vi "test-tagRouter.vi"() -> ()   [LabVIEW 2020]
uses:
  9c45d527-4fff-4982-a2e1-f8d778b02ec9.vi
  <userlib>/_NEVSTOP/Communicable State Machine(CSM)/AdvanceAPI/CSM - Break Down Multiple States String.vi
  <userlib>/_NEVSTOP/Communicable State Machine(CSM)/AdvanceAPI/CSM - Compact Multiple States.vi
  <userlib>/_NEVSTOP/Communicable State Machine(CSM)/AdvanceAPI/CSM - Revert Arguments-Safe String.vi
  <userlib>/_NEVSTOP/Communicable State Machine(CSM)/_Shared/Trim Single-line Text.vi
  <userlib>/_NEVSTOP/Communicable State Machine(CSM)/AdvanceAPI/CSM - Make String Arguments Safe.vi
  <userlib>/_NEVSTOP/Communicable State Machine(CSM)/AdvanceAPI/CSM - Keywords.vi
  <userlib>/_NEVSTOP/Communicable State Machine(CSM)/Utility/CSM Data Type String.vi
  <userlib>/_NEVSTOP/Communicable State Machine(CSM)/addons/MassData-Parameter/_support/FGV-MassData(lvlibp).vi
  CSM-TagRouter.lvlib
  <userlib>/_NEVSTOP/Communicable State Machine(CSM)/Communicable State Machine.lvlib
  <userlib>/_NEVSTOP/TagDB/TagDB.lvlib
panel:
  out "Data":variant[](array[variant])
  out "names":string[](array[string])
  in  "WaveformGen Settings":T1(array[cluster])=[{"sampling info"={"Fs"=1000.0, "#s"=1000.0}, "phase"=0.0, "amplitude"=1.0, "frequency"=10.0, "range"=1.0, "Type"=enum."Sine", "Waveform Name"="Waveform 0"}, {"sampling info"={"Fs"=1000.0, "#s"=1000.0}, "phase"=0.0, "amplitude"=1.0, "frequency"=10.0, "range"=1.0, "Type"=enum."Triangle", "Waveform Name"="Waveform 1"}, {"sampling info"={"Fs"=1000.0, "#s"=1000.0}, "phase"=0.0, "amplitude"=1.0, "frequency"=10.0, "range"=1.0, "Type"=enum."Sawtooth", "Waveform Name"="Waveform 2"}, {"sampling info"={"Fs"=1000.0, "#s"=1000.0}, "phase"=0.0, "amplitude"=1.0, "frequency"=10.0, "range"=1.0, "Type"=enum."Square", "Waveform Name"="Waveform 3"}]
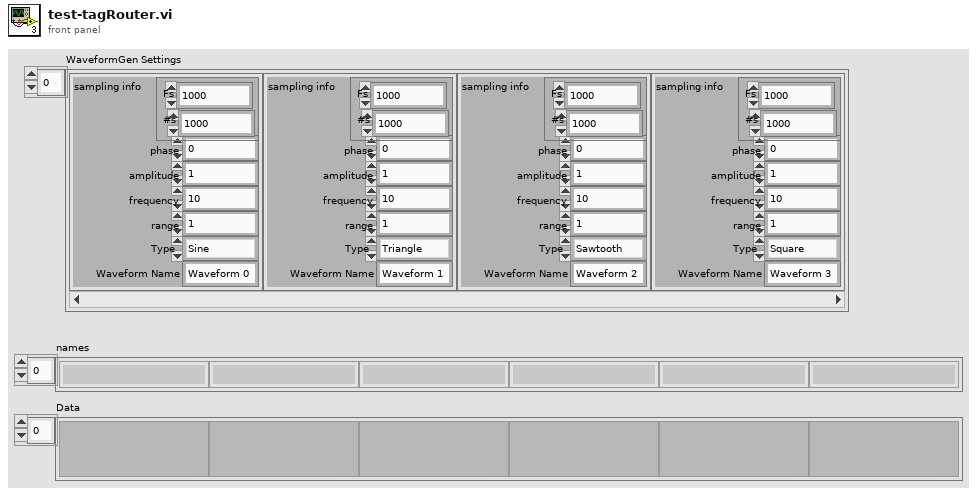
[diagram p1: front panel]
types:
  T1 = cluster{"sampling info":cluster{"Fs":dbl, "#s":dbl}, "phase":dbl, "amplitude":dbl, "frequency":dbl, "range":dbl, "Type":enum16{"Sine", "Triangle", "Sawtooth", "Square"}, "Waveform Name":string}[]
  T2 = enum32{"Invalid", "Standard", "Closed", "Hidden", "Minimized", "Maximized"}
  T3 = enum32{"invalid app kind", "Development System", "Run Time System", "Student Edition", "Embedded LabVIEW", "Evaluation", "Custom"}
  T4 = typedef "Communicable State Machine.lvlib/_CSM_Response Source Message.ctl" = cluster{"‘State":string, "’Arguments":string, "’Error":errorcluster}
  T5 = cluster{"Current VI Reference":refnum<vi>, "Close Panel on Exit?":bool}
  T6 = cluster{"Core":cluster{"Current VI Reference":refnum<vi>, "Close Panel on Exit?":bool}, "Your Boolean data":bool, "Your string data":string}
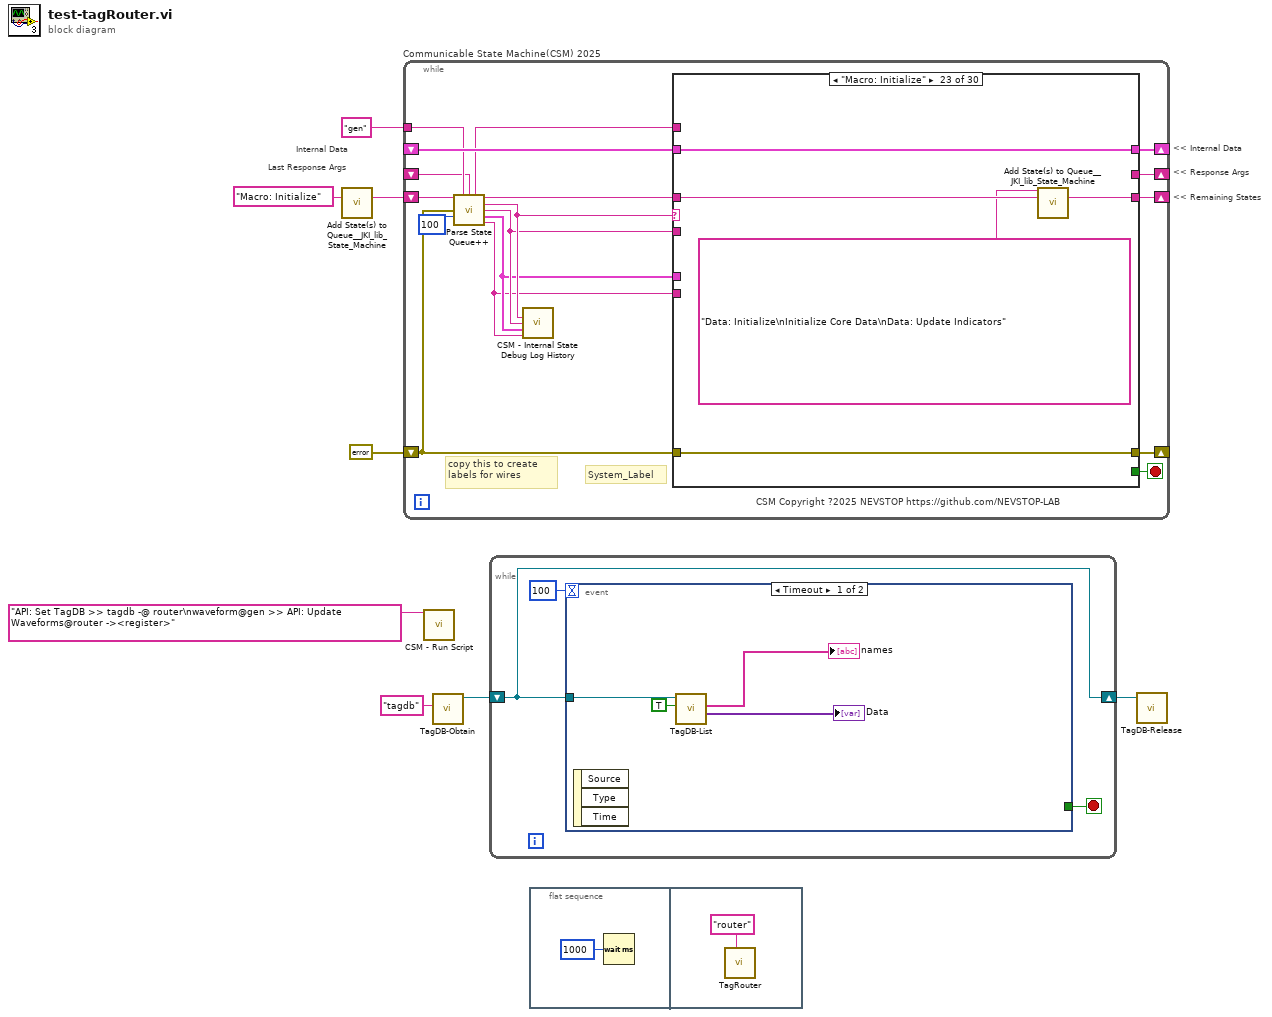
[diagram p0: block diagram]
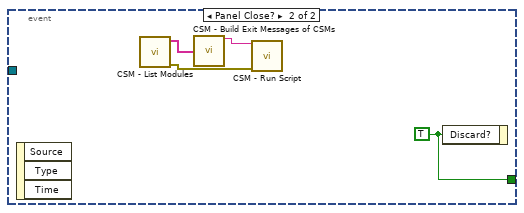
[diagram p2: hidden frame]
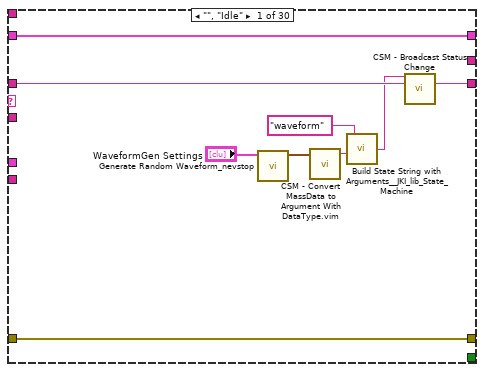
[diagram p3: hidden frame]
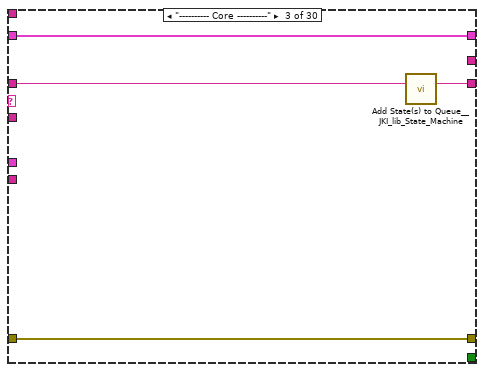
[diagram p5: hidden frame]
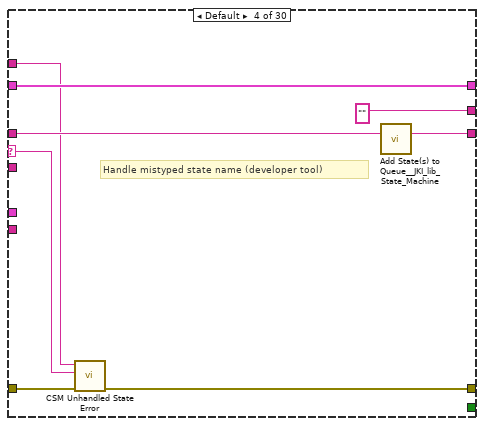
[diagram p6: hidden frame]
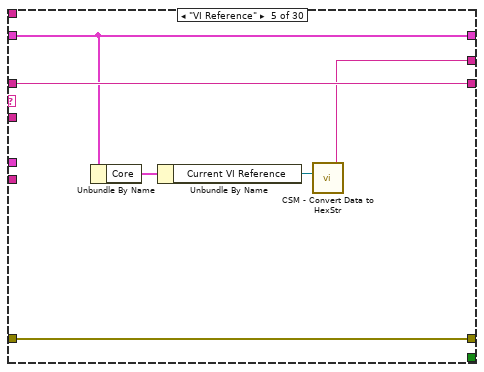
[diagram p7: hidden frame]
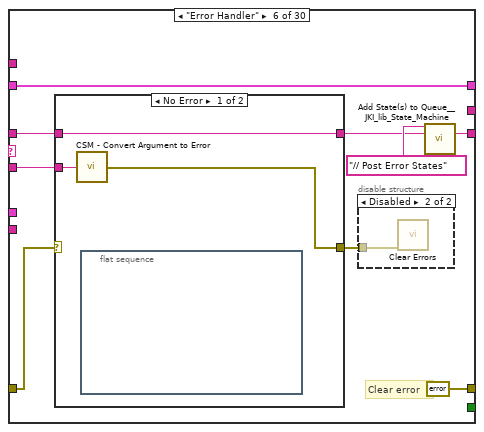
[diagram p8: hidden frame]
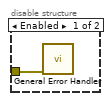
[diagram p9: hidden frame]
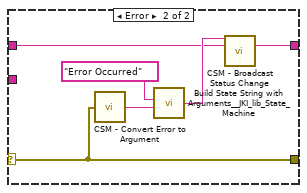
[diagram p10: hidden frame]
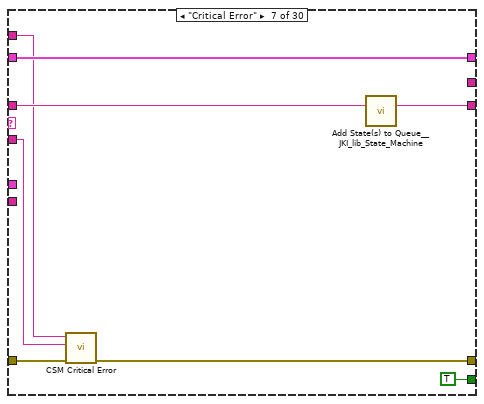
[diagram p11: hidden frame]
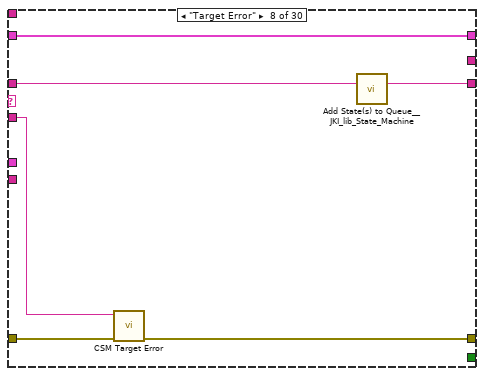
[diagram p12: hidden frame]
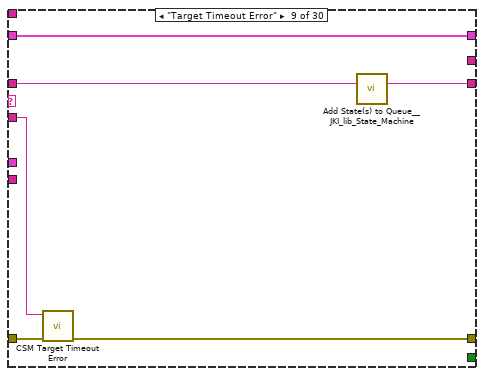
[diagram p13: hidden frame]
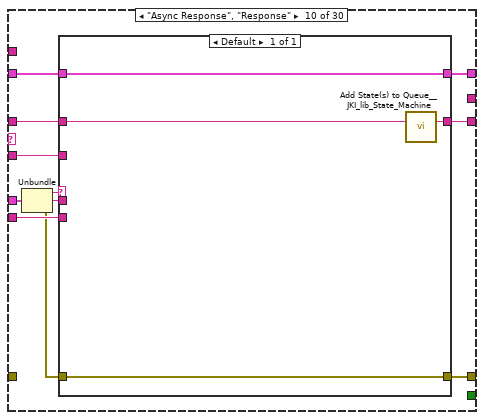
[diagram p14: hidden frame]
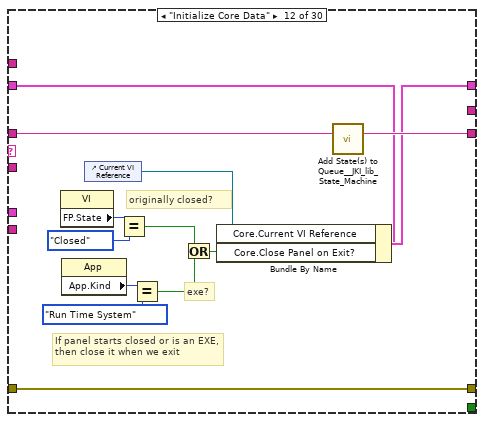
[diagram p16: hidden frame]
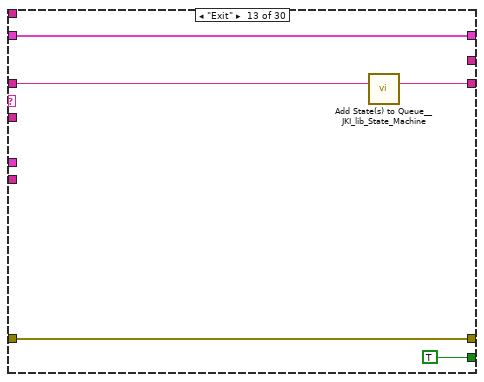
[diagram p17: hidden frame]
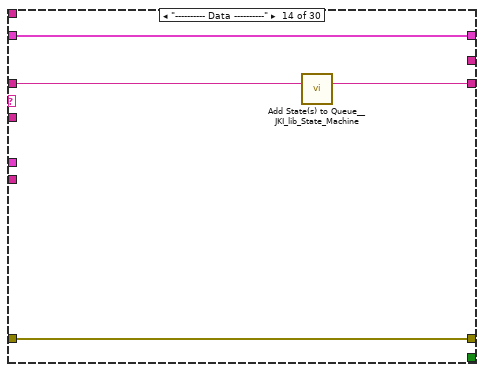
[diagram p18: hidden frame]
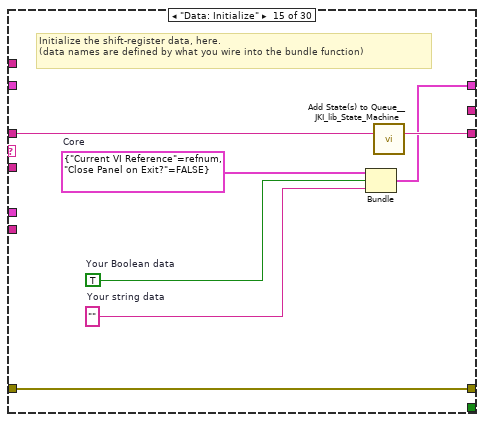
[diagram p19: hidden frame]
diagram:
  # "Last Response Args"
  # "Internal Data"
  # "<< Internal Data"
  # "<< Response Args"
  # "<< Remaining States"
  n1 = call <vilib>:"Add State(s) to Queue__JKI_lib_State_Machine.vi"("State(s) in (\"\")"="Macro: Initialize" ("Init State(\"Macro: Initialize\")")) -> ("States Out"=w5:string)  [unwired: 14 in]
  n2 = while "Communicable State Machine(CSM) 2025" {
    shift-right: [w20] -> _
    shift-left: _ -> [w19]
    shift-right: [w23] -> _
    shift-left: errorcluster {"status"=FALSE, "code"=0, "source"=""} ("error out") -> [w18]
    shift-right: [w22] -> _
    shift-left: w5 -> [w24]
    tunnel: "gen" ("Name (\"\" to Use UUID)") -> [w16]
    shift-right: [w17] -> _
    shift-left: _ -> [w10]
    stop <- w21 stop-if-true
    # "copy this to create labels for wires"
    # "System_Label"
    # "CSM Copyright ?2025 NEVSTOP https://github.com/NEVSTOP-LAB"
    n3 = call <userlib>:"Parse State Queue++.vi"("State Queue"=w24, "Name (\"\" to Use UUID)"=w16, "Response Arguments"=w10, "Previous Error"=w18, "Dequeue (1 ms)"=100 ("Timeout")) -> ("Name Used"=w11:string, "Remaining States"=w25:string, "Current State"=w15:string, "Arguments"=w14:string, "Additional Information"=w13:T4, "Source CSM"=w12:string)  [unwired: 5 in]
    n4 = call <userlib>:"CSM - Internal State Debug Log History.vi"("State"=w15, "Arguments (\"\")"=w14, ">> Response Source Message >>"=w13, "Source (\"\")"=w12) -> ()  [unwired: 11 in, 1 out]
    n5 = case shown="\"Macro: Initialize\"" w15 {
      selector: w15 -> [_ _ _ w44 _ _ _ _ _ _ _ _ _ _ _ _ _ _ _ _ _ _ _ _ _ _ _ _ _ _]
      tunnel: w25 -> [w31 w36 w41 w48 w54 w60 w81 w87 w93 w101 w112 w126 w131 w135 w142 w144 w151 w155 w159 w165 w180 w249 w254 w261 w263 w267 w272 w279 w283 w287]
      tunnel: w14 -> [_ _ _ _ _ w59 w77 w86 w91 w100 _ _ _ _ _ _ _ _ _ w160 w174 _ _ _ _ _ w270 _ _ _]
      tunnel: w19 -> [w32 w35 w38 w46 w53 w63 w82 w88 w94 w103 w111 w119 w129 w132 _ w143 w146 w152 w157 w163 w176 w246 w251 w258 w262 w266 w271 w276 w280 w284]
      tunnel: [w33 w37 w39 w42 w55 errorcluster {"status"=FALSE, "code"=0, "source"=""} ("error out") w78 w84 w90 w106 w113 w123 w128 w133 w139 w145 w147 w153 w156 w161 w177 w247 w252 w259 w264 w268 w273 w277 w281 w285] -> w23
      tunnel: w18 -> [w33 w37 w39 w49 w55 w61 w83 w85 w92 _ w113 w123 w128 w133 w139 w145 w148 w153 w156 w162 w178 w247 w252 w259 w264 w268 w273 w277 w281 w285]
      tunnel: [w34 w36 w40 w47 w54 w56 w80 w89 w95 w102 w112 w125 w130 w134 w141 w144 w150 w154 w158 w164 w179 w248 w253 w260 w263 w267 w272 w278 w282 w286] -> w22
      tunnel: [_ _ _ _ _ _ TRUE _ _ _ _ _ TRUE _ _ _ _ _ _ _ _ _ _ _ _ _ _ _ _ _] -> w21
      tunnel: [w32 w35 w38 w46 w53 w63 w82 w88 w94 w104 w111 w124 w129 w132 w140 w143 w146 w152 w157 w163 w176 w246 w251 w258 w262 w266 w271 w276 w280 w284] -> w20
      tunnel: w12 -> [_ _ _ _ _ _ _ _ _ w98 _ _ _ _ _ _ _ _ _ _ _ _ _ _ _ _ _ _ _ _]
      tunnel: w13 -> [_ _ _ _ _ _ _ _ _ w105 _ _ _ _ _ _ _ _ _ _ _ _ _ _ _ _ _ _ _ _]
      tunnel: [_ _ _ "" w50 _ _ _ _ _ _ _ _ _ _ _ _ _ _ _ _ _ _ _ _ "API1 Response" w269 _ _ _] -> w17
      tunnel: w11 -> [_ _ _ w43 _ _ w76 _ _ _ _ _ _ _ _ _ _ _ _ _ _ _ _ _ _ _ _ _ _ _]
      frame "", "Idle" {
        n6 = call <userlib>:"Generate Random Waveform_nevstop.vi"("WaveformGen Settings"="WaveformGen Settings") -> ("Waveforms"=w29:waveform(dbl)[])  [unwired: 9 in, 1 out]
        n7 = call "CSM - Convert MassData to Argument With DataType.vim"("Data"=w29) -> ("MassData Argument"=w28:string)  [unwired: 7 in, 1 out]
        n8 = call <vilib>:"Build State String with Arguments__JKI_lib_State_Machine.vi"("Arguments (\"\")"=w28, "State"="waveform") -> ("State with Arguments"=w26:string)  [unwired: 4 in]
        n9 = call <userlib>:"CSM - Broadcast Status Change.vi"("Status With Arguments"=w26, "State Queue"=w31) -> ("Remaining States"=w34:string)  [unwired: 13 in]
      }
      frame "CSM Documentation" {
      }
      frame "---------- Core ----------" {
        n10 = call <vilib>:"Add State(s) to Queue__JKI_lib_State_Machine.vi"("State(s) in (\"\")"=w41) -> ("States Out"=w40:string)  [unwired: 14 in]
      }
      frame Default {
        # "Handle mistyped state name (developer tool)"
        n11 = call <userlib>:"CSM Unhandled State Error.vi"("error in (no error)"=w49, "Undefined State"=w44, "CSM Name"=w43) -> ("error out"=w42:errorcluster)  [unwired: 8 in]
        n12 = call <vilib>:"Add State(s) to Queue__JKI_lib_State_Machine.vi"("State(s) in (\"\")"=w48) -> ("States Out"=w47:string)  [unwired: 14 in]
      }
      frame "VI Reference" {
        n13 = Unbundle By Name(w53) -> ("Core"=w52:T5)
        n14 = Unbundle By Name(w52) -> ("Current VI Reference"=w51:refnum<vi>)
        n15 = call <userlib>:"CSM - Convert Data to HexStr.vi"("Variant"=w51) -> ("HEX String (0-9,A-F)"=w50:string)  [unwired: 8 in]
      }
      frame "Error Handler" {
        # "Clear error"
        n16 = case shown="No Error" w61 {
          selector: w61 -> [_ w70]
          tunnel: [w69 w72] -> w57
          tunnel: w60 -> [w69 w71]
          tunnel: w59 -> [w68 _]
          tunnel: [w67 w70] -> w62
          frame No Error {
            n17 = call <userlib>:"CSM - Convert Argument to Error.vi"("Argument"=w68) -> ("Error"=w67:errorcluster)  [unwired: 4 in]
            n18 = flat-sequence {
              frame #0 {
              }
            }
          }
          frame Error {
            n19 = call <userlib>:"CSM - Convert Error to Argument.vi"("Error"=w70) -> ("Argument"=w74:string)  [unwired: 4 in]
            n20 = call <vilib>:"Build State String with Arguments__JKI_lib_State_Machine.vi"("Arguments (\"\")"=w74, "State"="Error Occurred" ("Status with Arguments")) -> ("State with Arguments"=w73:string)  [unwired: 4 in]
            n21 = call <userlib>:"CSM - Broadcast Status Change.vi"("Status With Arguments"=w73, "State Queue"=w71) -> ("Remaining States"=w72:string)  [unwired: 13 in]
          }
        }
        n22 = disable-structure shown="Disabled" {
          disable-tunnel: w62 -> [w65 w66]
          frame Enabled {
            n23 = call <vilib>:"General Error Handler.vi"("error in (no error)"=w65) -> ()  [unwired: 10 in, 5 out]
          }
          frame Disabled {
            n24 = call <vilib>:"Clear Errors.vi"("error in (no error)"=w66) -> ()  [unwired: 5 in, 2 out]
          }
        }
        n25 = call <vilib>:"Add State(s) to Queue__JKI_lib_State_Machine.vi"("State(s) in Front (\"\")"="// Post Error States", "State(s) in (\"\")"=w57) -> ("States Out"=w56:string)  [unwired: 13 in]
      }
      frame "Critical Error" {
        n26 = call <userlib>:"CSM Critical Error.vi"("error in (no error)"=w83, "Arugments (As Reason)"=w77, "CSM Name"=w76) -> ("error out"=w78:errorcluster)  [unwired: 8 in]
        n27 = call <vilib>:"Add State(s) to Queue__JKI_lib_State_Machine.vi"("State(s) in (\"\")"=w81) -> ("States Out"=w80:string)  [unwired: 14 in]
      }
      frame "Target Error" {
        n28 = call <userlib>:"CSM Target Error.vi"("error in (no error)"=w85, "Arguments (As CSM Name)"=w86) -> ("error out"=w84:errorcluster)  [unwired: 9 in]
        n29 = call <vilib>:"Add State(s) to Queue__JKI_lib_State_Machine.vi"("State(s) in (\"\")"=w87) -> ("States Out"=w89:string)  [unwired: 14 in]
      }
      frame "Target Timeout Error" {
        n30 = call <userlib>:"CSM Target Timeout Error.vi"("error in (no error)"=w92, "Arguments (As CSM Name)"=w91) -> ("error out"=w90:errorcluster)  [unwired: 9 in]
        n31 = call <vilib>:"Add State(s) to Queue__JKI_lib_State_Machine.vi"("State(s) in (\"\")"=w93) -> ("States Out"=w95:string)  [unwired: 14 in]
      }
      frame "Async Response", "Response" {
        n32 = Unbundle(w105) -> ("‘State"=w99:string, "’Arguments"=w97:string, "’Error"=w96:errorcluster)
        n33 = case shown="Default" w99 {
          tunnel: [w110] -> w106
          tunnel: w96 -> [w110]
          tunnel: [w109] -> w104
          tunnel: w103 -> [w109]
          tunnel: [w107] -> w102
          tunnel: w101 -> [w108]
          tunnel: w100 -> [_]
          tunnel: w98 -> [_]
          tunnel: w97 -> [_]
          frame Default {
            n34 = call <vilib>:"Add State(s) to Queue__JKI_lib_State_Machine.vi"("State(s) in (\"\")"=w108) -> ("States Out"=w107:string)  [unwired: 14 in]
          }
        }
      }
      frame "Async Message Posted" {
      }
      frame "Initialize Core Data" {
        # "originally closed?"
        # "exe?"
        # "If panel starts closed or is an EXE, then close it when we exit"
        n35 = property class="VI"() -> ("FP.State"=w116:T2)  [unwired: 2 in, 2 out]
        n36 = property class="App"() -> ("App.Kind"=w122:T3)  [unwired: 2 in, 2 out]
        n37 = control-ref of="Current VI Reference"() -> (w117:refnum<vi>)
        n38 = Equal?(x=w116, y=T2."Closed" ("Front Panel Window:State")) -> (x = y?=w114:bool)
        n39 = Equal?(x=w122, y=T3."Run Time System" ("Application:Kind")) -> (x = y?=w120:bool)
        n40 = Or(x=w114, y=w120) -> (x .or. y?=w118:bool)
        n41 = Bundle By Name(cluster=w119, "Core.Current VI Reference"=w117, "Core.Close Panel on Exit?"=w118) -> (w124:T6)
        n42 = call <vilib>:"Add State(s) to Queue__JKI_lib_State_Machine.vi"("State(s) in (\"\")"=w126) -> ("States Out"=w125:string)  [unwired: 14 in]
      }
      frame "Exit" {
        n43 = call <vilib>:"Add State(s) to Queue__JKI_lib_State_Machine.vi"("State(s) in (\"\")"=w131) -> ("States Out"=w130:string)  [unwired: 14 in]
      }
      frame "---------- Data ----------" {
        n44 = call <vilib>:"Add State(s) to Queue__JKI_lib_State_Machine.vi"("State(s) in (\"\")"=w135) -> ("States Out"=w134:string)  [unwired: 14 in]
      }
      frame "Data: Initialize" {
        w136 = T5 {"Current VI Reference"=refnum, "Close Panel on Exit?"=FALSE}  # Core
        w138 = TRUE  # Your Boolean data
        w137 = ""  # Your string data
        # "Initialize the shift-register data, here.\n(data names are defined by what you wire into the bundle function)"
        n45 = Bundle("Core"=w136, "Your Boolean data"=w138, "Your string data"=w137) -> (w140:T6)  [unwired: 1 in]
        n46 = call <vilib>:"Add State(s) to Queue__JKI_lib_State_Machine.vi"("State(s) in (\"\")"=w142) -> ("States Out"=w141:string)  [unwired: 14 in]
      }
      frame "Data: Update Indicators" {
      }
      frame "Data: Cleanup" {
        # "Cleanup any data and references, here.\n(this is called automatically, by the Macro: Exit)"
        n47 = Unbundle By Name(w146) -> ("Core.Current VI Reference"=w149:refnum<vi>)
        n48 = Close Reference(reference=w149, error in (no error)=w148) -> (error out=w147:errorcluster)
        n49 = call <vilib>:"Add State(s) to Queue__JKI_lib_State_Machine.vi"("State(s) in (\"\")"=w151) -> ("States Out"=w150:string)  [unwired: 14 in]
      }
      frame "---------- UI ----------" {
        n50 = call <vilib>:"Add State(s) to Queue__JKI_lib_State_Machine.vi"("State(s) in (\"\")"=w155) -> ("States Out"=w154:string)  [unwired: 14 in]
      }
      frame "UI: Initialize" {
        n51 = call <vilib>:"Add State(s) to Queue__JKI_lib_State_Machine.vi"("State(s) in (\"\")"=w159) -> ("States Out"=w158:string)  [unwired: 14 in]
      }
      frame "UI: Cursor Set" {
        # "Argument"
        n52 = disable-structure shown="TARGET_TYPE!=Windows" {
          disable-tunnel: w162 -> [w168 w173]
          disable-tunnel: [w167 w173] -> w161
          disable-tunnel: w160 -> [w166 _]
          frame condition #0 (active) {
            n53 = case shown="\"Idle\", Default" w166 {
              tunnel: w168 -> [w170 w172]
              tunnel: [w169 w171] -> w167
              frame "Idle", Default {
                n54 = call <vilib>:"Unset Busy.vi"("error in (no error)"=w170) -> ("error out"=w169:errorcluster)  [unwired: 10 in]
              }
              frame "Busy" {
                n55 = call <vilib>:"Set Busy.vi"("error in (no error)"=w172) -> ("error out"=w171:errorcluster)  [unwired: 9 in, 1 out]
              }
            }
          }
          frame condition #1 {
          }
        }
        n56 = call <vilib>:"Add State(s) to Queue__JKI_lib_State_Machine.vi"("State(s) in (\"\")"=w165) -> ("States Out"=w164:string)  [unwired: 14 in]
      }
      frame "UI: Front Panel State" {
        # "Argument"
        n57 = Unbundle By Name(w176) -> ("Core.Current VI Reference"=w175:refnum<vi>)
        n58 = call <vilib>:"Add State(s) to Queue__JKI_lib_State_Machine.vi"("State(s) in (\"\")"=w180) -> ("States Out"=w179:string)  [unwired: 14 in]
        n59 = case shown="\"Close\", \"Closed\"" w174 {
          tunnel: w178 -> [w186 w201 w212 w225 w238]
          tunnel: [w188 w202 w214 w227 w240] -> w177
          tunnel: w175 -> [w187 w199 w213 w226 w239]
          frame "Open", "Standard", Default {
            w181 = T2."Standard" ("State")
            n60 = property class="VI"(reference=w187, error in=w186) -> (reference out=w184:refnum<vi>, error out=w185:errorcluster, "FP.State"=w183:T2)
            n61 = Not Equal?(x=w183, y=w181) -> (x != y?=w182:bool)
            n62 = case shown="True" w182 {
              tunnel: [w192 w194] -> w188
              tunnel: w185 -> [w191 w194]
              tunnel: w184 -> [w190 _]
              tunnel: w181 -> [w189 _]
              frame True {
                n63 = invoke class="VI" method="FP.Open"(reference=w190, error in=w191, "Activate"=TRUE, "State"=w189) -> (error out=w192:errorcluster)  [unwired: 1 in, 4 out]
              }
              frame False {
              }
            }
          }
          frame "Close", "Closed" {
            n64 = property class="VI"(reference=w199, error in=w201) -> (reference out=w198:refnum<vi>, error out=w200:errorcluster, "FP.State"=w196:T2)
            n65 = Not Equal?(x=w196, y=T2."Closed" ("Front Panel Window:State")) -> (x != y?=w195:bool)
            n66 = case shown="False" w195 {
              tunnel: [w203 w206] -> w202
              tunnel: w200 -> [w203 w205]
              tunnel: w198 -> [_ w204]
              frame False {
              }
              frame True {
                n67 = invoke class="VI" method="FP.Close"(reference=w204, error in=w205) -> (error out=w206:errorcluster)  [unwired: 1 in, 2 out]
              }
            }
          }
          frame "Hidden", "Hide" {
            w207 = T2."Hidden" ("State")
            n68 = property class="VI"(reference=w213, error in=w212) -> (reference out=w210:refnum<vi>, error out=w211:errorcluster, "FP.State"=w209:T2)
            n69 = Not Equal?(x=w209, y=w207) -> (x != y?=w208:bool)
            n70 = case shown="True" w208 {
              tunnel: [w218 w219] -> w214
              tunnel: w211 -> [w217 w219]
              tunnel: w210 -> [w216 _]
              tunnel: w207 -> [w215 _]
              frame True {
                n71 = invoke class="VI" method="FP.Open"(reference=w216, error in=w217, "State"=w215) -> (error out=w218:errorcluster)  [unwired: 2 in, 4 out]
              }
              frame False {
              }
            }
          }
          frame "Minimize", "Minimized" {
            w220 = T2."Minimized" ("State")
            n72 = property class="VI"(reference=w226, error in=w225) -> (reference out=w223:refnum<vi>, error out=w224:errorcluster, "FP.State"=w222:T2)
            n73 = Not Equal?(x=w222, y=w220) -> (x != y?=w221:bool)
            n74 = case shown="True" w221 {
              tunnel: [w231 w232] -> w227
              tunnel: w224 -> [w230 w232]
              tunnel: w223 -> [w229 _]
              tunnel: w220 -> [w228 _]
              frame True {
                n75 = invoke class="VI" method="FP.Open"(reference=w229, error in=w230, "State"=w228) -> (error out=w231:errorcluster)  [unwired: 2 in, 4 out]
              }
              frame False {
              }
            }
          }
          frame "Maximize", "Maximized" {
            w233 = T2."Maximized" ("State")
            n76 = property class="VI"(reference=w239, error in=w238) -> (reference out=w236:refnum<vi>, error out=w237:errorcluster, "FP.State"=w235:T2)
            n77 = Not Equal?(x=w235, y=w233) -> (x != y?=w234:bool)
            n78 = case shown="True" w234 {
              tunnel: [w244 w245] -> w240
              tunnel: w237 -> [w243 w245]
              tunnel: w236 -> [w242 _]
              tunnel: w233 -> [w241 _]
              frame True {
                n79 = invoke class="VI" method="FP.Open"(reference=w242, error in=w243, "State"=w241) -> (error out=w244:errorcluster)  [unwired: 2 in, 4 out]
              }
              frame False {
              }
            }
          }
        }
      }
      frame "---------- Macro ----------" {
        n80 = call <vilib>:"Add State(s) to Queue__JKI_lib_State_Machine.vi"("State(s) in (\"\")"=w249) -> ("States Out"=w248:string)  [unwired: 14 in]
      }
      frame "Macro: Initialize" {
        n81 = call <vilib>:"Add State(s) to Queue__JKI_lib_State_Machine.vi"("State(s) in Front (\"\")"="Data: Initialize\nInitialize Core Data\nData: Update Indicators", "State(s) in (\"\")"=w254) -> ("States Out"=w253:string)  [unwired: 13 in]
      }
      frame "Macro: Exit" {
        n82 = call <vilib>:"Add State(s) to Queue__JKI_lib_State_Machine.vi"("State(s) in Front (\"\")"="//Exit Sub-Modules ", "State(s) at Back (\"\")"="Data: Cleanup\nExit") -> ("States Out"=w256:string)  [unwired: 13 in]
        n83 = call <vilib>:"Add State(s) to Queue__JKI_lib_State_Machine.vi"("State(s) in Front (\"\")"=w256, "State(s) in (\"\")"=w261) -> ("States Out"=w260:string)  [unwired: 13 in]
      }
      frame "---------- API ----------" {
      }
      frame "API: API1" {
      }
      frame "API: API2" {
        # "unpack Hex String  to Variant\nif complex parameter is needed."
        n84 = call <userlib>:"CSM - Convert HexStr to Data.vi"("HEX String"=w270) -> ()  [unwired: 7 in, 2 out]
        n85 = disable-structure shown="Disabled" {
          disable-tunnel: [w274 "API2 Response"] -> w269
          frame Disabled {
            # "pack variant to hexstr \nif complex response is needed."
            # "complex Response"
            n86 = call <userlib>:"CSM - Convert Data to HexStr.vi"() -> ("HEX String (0-9,A-F)"=w274:string)  [unwired: 9 in]
          }
          frame Enabled {
          }
        }
      }
      frame "---------- Action ----------" {
        n87 = call <vilib>:"Add State(s) to Queue__JKI_lib_State_Machine.vi"("State(s) in (\"\")"=w279) -> ("States Out"=w278:string)  [unwired: 14 in]
      }
      frame "Action: action1" {
        n88 = call <vilib>:"Add State(s) to Queue__JKI_lib_State_Machine.vi"("State(s) in (\"\")"=w283) -> ("States Out"=w282:string)  [unwired: 14 in]
      }
      frame "Action: action2" {
        n89 = call <vilib>:"Add State(s) to Queue__JKI_lib_State_Machine.vi"("State(s) in (\"\")"=w287) -> ("States Out"=w286:string)  [unwired: 14 in]
      }
    }
  }
  n90 = call <userlib>:"CSM - Run Script.vi"("CSM Scripts"="API: Set TagDB >> tagdb -@ router\nwaveform@gen >> API: Update Waveforms@router -><register>" ("States With Replace Token")) -> ()  [unwired: 12 in, 3 out]
  n91 = call <userlib>:"TagDB-Obtain.vi"("name (unnamed)"="tagdb") -> ("TagDB"=w2:refnum<k1>)  [unwired: 4 in, 2 out]
  n92 = while {
    shift-right: [w288] -> w1
    shift-left: w2 -> [w288]
    stop <- w290 stop-if-true
    n93 = event shown="[0] Timeout" {
      selector: _ -> [_ _]
      dyn-events: _ -> [_ _]
      timeout: 100 -> [_ _]
      tunnel: [_ w298] -> w290
      tunnel: w288 -> [w294 _]
      event Timeout {
        n94 = event-data() -> ()  [unwired: 1 in, 3 out]
        n95 = call <userlib>:"TagDB-List.vi"("with Data?(F)"=TRUE, "TagDB"=w294) -> ("Data"=→"Data":variant[], "names"=→"names":string[])  [unwired: 6 in, 2 out]
      }
      event Panel Close? {
        w298 = TRUE ("Discard?")
        n96 = event-data() -> ()  [unwired: 1 in, 3 out]
        n97 = call <userlib>:"CSM - List Modules.vi"() -> ("error out"=w295:errorcluster, "Module Names"=w297:string[])  [unwired: 10 in]
        n98 = call <userlib>:"CSM - Build Exit Messages of CSMs.vi"("CSMs"=w297) -> ("States"=w296:string)  [unwired: 14 in]
        n99 = call <userlib>:"CSM - Run Script.vi"("CSM Scripts"=w296, "error in (no error)"=w295) -> ()  [unwired: 11 in, 3 out]
        n100 = event-data("Discard?"=w298) -> ()  [unwired: 1 in, 1 out]
      }
    }
  }
  n101 = flat-sequence {
    frame #0 {
      n102 = Wait (ms)(milliseconds to wait=u32 1000) -> ()  [unwired: 1 out]
    }
    frame #1 {
      n103 = call "TagRouter.vi"("Name(\"\" to use uuid)"="router" ("Name(\"\" to use uuid)")) -> ()  [unwired: 11 in]
    }
  }
  n104 = call <userlib>:"TagDB-Release.vi"("TagDB"=w1) -> ()  [unwired: 10 in, 1 out]
